vi "GetUser.vi"(11 "权限":string(combo)="QX01") -> (0 "员工姓名":string, 1 "权限":bool, 2 "输入员工ID":string)   [LabVIEW 2013]
uses:
  <vilib>/Utility/error.llb/whitespace.ctl
panel:
  in  "error in (no error)":errorcluster
  out "error out":errorcluster
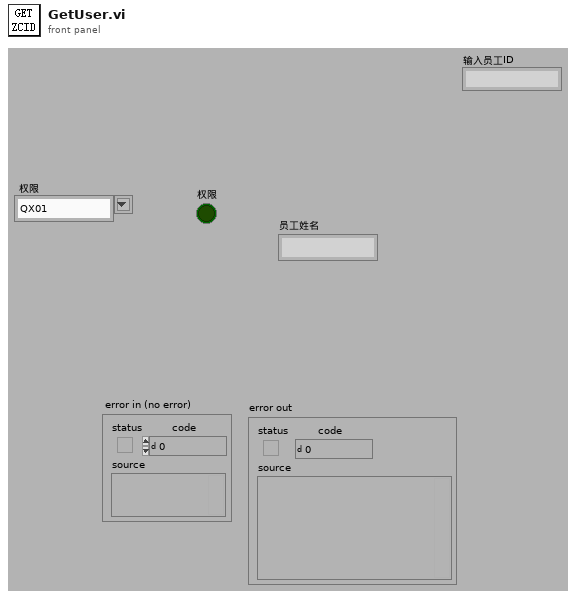
[diagram p1: front panel]
types:
  T1 = typedef "whitespace.ctl" = u16
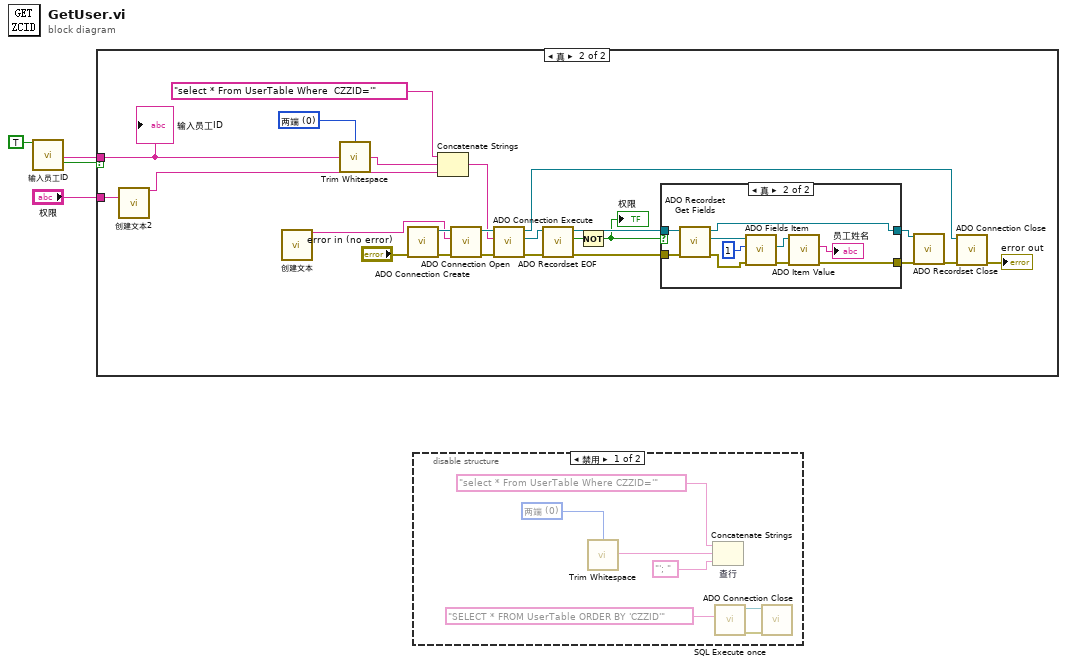
[diagram p0: block diagram]
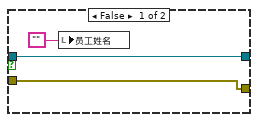
[diagram p3: hidden frame]
diagram:
  n1 = call "输入员工ID.vi"("Enable"=TRUE) -> ("输入员工ID"=w4:string, "确定"=w2:bool)  [unwired: 16 in, 1 out]
  n2 = case shown="真" w2 {
    tunnel: w4 -> [_ w7]
    tunnel: "权限" -> [_ w5]
    frame False {
    }
    frame True {
      w20 = T1 0 items=["两端", "字符串首端", "字符串末端"] ("location (both)")
      n3 = call "创建文本2"("权限"=w5) -> ("Result"=w6:string)  [unwired: 13 in, 1 out]
      n4 = call "创建文本"() -> ("Result"=w9:string)  [unwired: 14 in, 1 out]
      n5 = call <vilib>:"Trim Whitespace.vi"("string"=w7, "location (both)"=w20) -> ("trimmed string"=w21:string)
      n6 = call "ADO Connection Create.vi"("error in (no error)"="error in (no error)") -> ("error out"=w27:errorcluster, "ADODB._Connection Out"=w28:refnum<k7>)  [unwired: 9 out]
      n7 = Concatenate Strings ("查位置")("select * From UserTable Where  CZZID='" ("字符串 2"), w21, w6) -> (w10:string)
      n8 = call "ADO Connection Open.vi"("error in (no error)"=w27, "ConnectionString"=w9, "ADODB._Connection In"=w28) -> ("error out"=w26:errorcluster, "ADODB._Connection Out"=w11:refnum<k7>)  [unwired: 7 out]
      n9 = call "ADO Connection Execute.vi"("error in (no error)"=w26, "CommandText"=w10, "ADODB._Connection In"=w11) -> ("error out"=w24:errorcluster, "RecordSet"=w25:refnum<k7>, "ADODB._Connection Out"=w12:refnum<k7>)  [unwired: 6 out]
      n10 = call "ADO Recordset EOF.vi"("error in (no error)"=w24, "ADODB._Recordset In"=w25) -> ("error out"=w16:errorcluster, "EOF"=w13:bool, "ADODB._Recordset Out"=w17:refnum<k7>)  [unwired: 7 out]
      n11 = Not(x=w13) -> (.not. x?=w8:bool)
      "权限" <- w8
      n12 = case shown="真" w8 {
        tunnel: w17 -> [w30 w41]
        tunnel: w16 -> [w31 w40]
        tunnel: [w30 w39] -> w15
        tunnel: [w31 w33] -> w14
        frame False {
          n13 = local write "员工姓名"("") -> ()
        }
        frame True {
          n14 = call "ADO Recordset Get Fields.vi"("error in (no error)"=w40, "ADODB._Recordset In"=w41) -> ("error out"=w32:errorcluster, "Fields Out"=w38:refnum<k7>, "ADODB._Recordset Out"=w39:refnum<k7>)  [unwired: 7 out]
          n15 = call "ADO Fields Item.vi"("error in (no error)"=w32, "Index"=1, "Fields In"=w38) -> ("error out"=w36:errorcluster, "Item Out"=w35:refnum<k7>)  [unwired: 7 out]
          n16 = call "ADO Item Value.vi"("error in (no error)"=w36, "Item In"=w35) -> ("error out"=w33:errorcluster, "Value"=→"员工姓名":string)  [unwired: 8 out]
        }
      }
      n17 = call "ADO Recordset Close.vi"("ADODB._Recordset In"=w15, "error in (no error)"=w14) -> ("error out"=w23:errorcluster)  [unwired: 17 out]
      n18 = call "ADO Connection Close.vi"("error in (no error)"=w23, "ADODB._Connection In"=w12) -> ("error out"=→"error out":errorcluster)  [unwired: 9 out]
      "输入员工ID" <- w7
    }
  }
  n19 = disable-structure shown="禁用" {
    frame Disabled {
      w45 = T1 0 items=["两端", "字符串首端", "字符串末端"] ("location (both)")
      n20 = call <vilib>:"Trim Whitespace.vi"("location (both)"=w45) -> ("trimmed string"=w44:string)  [unwired: 1 in]
      n21 = Concatenate Strings "查行"("select * From UserTable Where CZZID='" ("字符串 2"), w44, "'; " ("字符串 2")) -> ()  [unwired: 1 out]
      n22 = call "SQL Execute once.vi"("Command Text"="SELECT * FROM UserTable ORDER BY 'CZZID'") -> ("error out"=w48:errorcluster, "ADODB._Connection Out"=w47:refnum<k7>)  [unwired: 3 in, 6 out]
      n23 = call "ADO Connection Close.vi"("error in (no error)"=w48, "ADODB._Connection In"=w47) -> ()  [unwired: 10 out]
    }
    frame Enabled {
    }
  }
